vi "string_right.vi"(10 "length":i32=4, 11 "string":string) -> (3 "to":string)   [LabVIEW 2011]
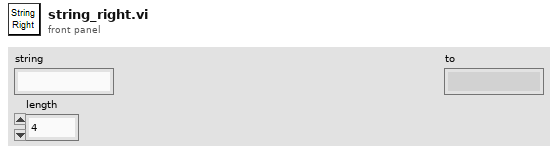
[diagram p1: front panel]
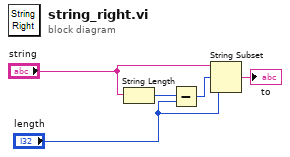
[diagram p0: block diagram]
diagram:
  n1 = String Length(string="string") -> (length=w5:i32)
  n2 = Subtract(x=w5, y="length") -> (x-y=w4:i32)
  n3 = String Subset(string="string", offset (0)=w4, length (rest)="length") -> (substring=→"to":string)
